vi "跑马灯.vi"() -> ()   [LabVIEW 2022 SP3]
panel:
  in  "?":bool
  in  "闪烁间隔（ms）":dbl(slide) scale=0.0..500.0
  out "?":bool
  out "?":bool
  out "?":bool
  out "?":bool
  out "?":bool
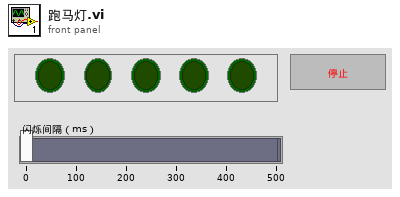
[diagram p1: front panel]
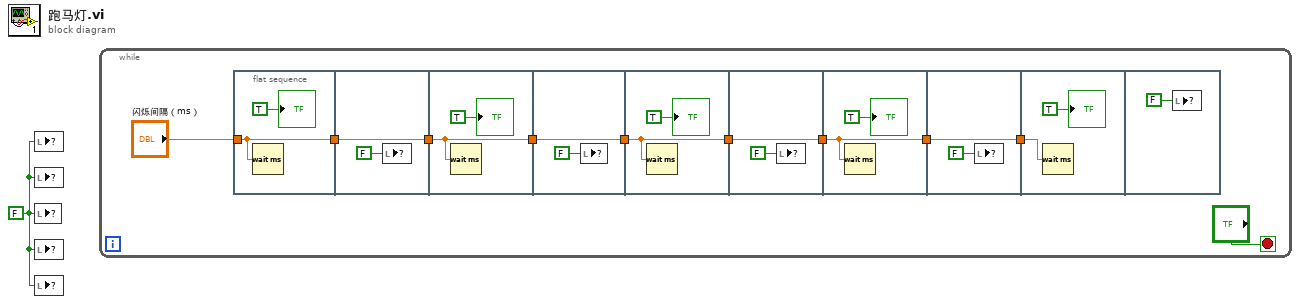
[diagram p0: block diagram]
diagram:
  w1 = FALSE
  n1 = local write item#4(w1) -> ()
  n2 = local write item#2(w1) -> ()
  n3 = local write item#1(w1) -> ()
  n4 = local write item#?(w1) -> ()
  n5 = local write item#3(w1) -> ()
  n6 = while {
    stop <- "?" stop-if-true
    n7 = flat-sequence {
      tunnel: "闪烁间隔（ms）" -> [w13]
      tunnel: [w13] -> w11
      tunnel: w11 -> [w15]
      tunnel: [w15] -> w10
      tunnel: w10 -> [w17]
      tunnel: [w17] -> w9
      tunnel: w9 -> [w19]
      tunnel: [w19] -> w8
      tunnel: w8 -> [w21]
      tunnel: [w21] -> w7
      tunnel: w7 -> [w23]
      tunnel: [w23] -> w6
      tunnel: w6 -> [w25]
      tunnel: [w25] -> w5
      tunnel: w5 -> [w27]
      tunnel: [w27] -> w4
      tunnel: w4 -> [w29]
      frame #0 {
        n8 = Wait (ms)(milliseconds to wait=w13) -> ()  [unwired: 1 out]
        "?" <- TRUE
      }
      frame #1 {
        n9 = local write item#?(FALSE) -> ()
      }
      frame #2 {
        n10 = Wait (ms)(milliseconds to wait=w17) -> ()  [unwired: 1 out]
        "?" <- TRUE
      }
      frame #3 {
        n11 = local write item#1(FALSE) -> ()
      }
      frame #4 {
        n12 = Wait (ms)(milliseconds to wait=w21) -> ()  [unwired: 1 out]
        "?" <- TRUE
      }
      frame #5 {
        n13 = local write item#2(FALSE) -> ()
      }
      frame #6 {
        n14 = Wait (ms)(milliseconds to wait=w25) -> ()  [unwired: 1 out]
        "?" <- TRUE
      }
      frame #7 {
        n15 = local write item#3(FALSE) -> ()
      }
      frame #8 {
        n16 = Wait (ms)(milliseconds to wait=w29) -> ()  [unwired: 1 out]
        "?" <- TRUE
      }
      frame #9 {
        n17 = local write item#4(FALSE) -> ()
      }
    }
  }
